vi "图片创建与保存.vi"() -> ()   [LabVIEW 2018]
panel:
  in  "?":bool
  out "图像创建":bool
  in  "Read Path":path
  out "error out":errorcluster
  out "Image":T1(plugin-control)
  in  "Image Type":T2 items=["Grayscale (U8)", "Grayscale (I16)", "Grayscale (SGL)", "Complex (CSG)", "RGB (U32)", "HSL (U32)", "RGB (U64)", "Grayscale (U16)"]
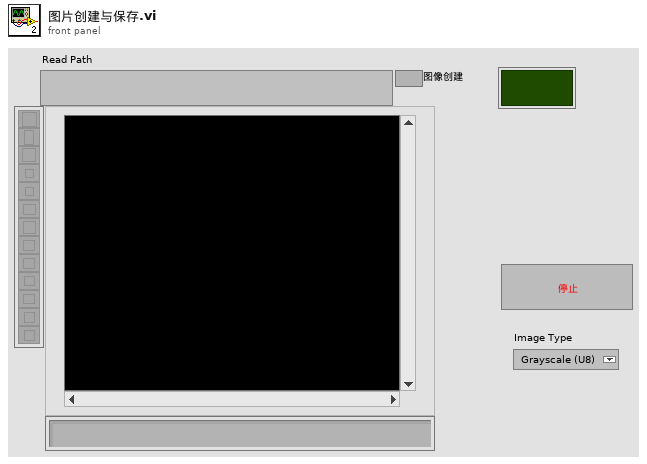
[diagram p1: front panel]
types:
  T1 = typedef "IMAQ Image.ctl" = refnum<image>
  T2 = typedef "Image Type" = u32
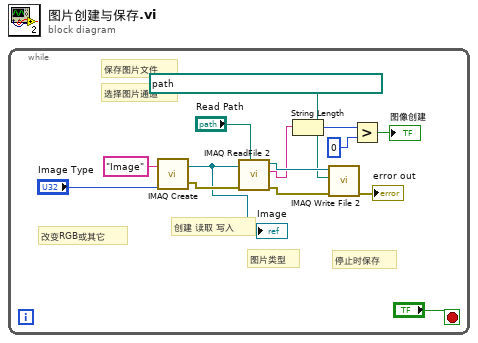
[diagram p0: block diagram]
diagram:
  n1 = while {
    stop <- "?" stop-if-true
    # "停止时保存"
    # "保存图片文件"
    # "选择图片通道"
    # "改变RGB或其它"
    # "图片类型"
    # "创建 读取 写入"
    n2 = call "IMAQ Create"("Image Name"="Image", "Image Type"="Image Type") -> ("New Image"=w9:T1, "error out"=w13:errorcluster)  [unwired: 3 in]
    "Image" <- w9
    n3 = call "IMAQ ReadFile 2"("File Path"="Read Path", "error in (no error)"=w13, "Image"=w9) -> ("error out"=w12:errorcluster, "File Type out"=w5:string, "Image Out"=w14:T1)  [unwired: 4 in, 2 out]
    n4 = String Length(string=w5) -> (length=w4:i32)
    n5 = call-poly "IMAQ Write File 2"("error in (no error)"=w12, "File Path"=path "D:/Labviewprogram/视觉/Iamge1.png", "Image"=w14) -> ("error out"=→"error out":errorcluster)  [unwired: 7 in, 1 out]
    n6 = Greater?(x=w4, y=0) -> (0:→"图像创建":bool)
  }
